vi "Practice with Arrays.vi"() -> ()   [LabVIEW 2016]
panel:
  out "y":dbl[](array[numeric])
  out "x-y":dbl[](array[numeric])
  out "x":dbl[](array[numeric])
  in  "Input Array":dbl[](array[numeric])
  in  "Input element":dbl
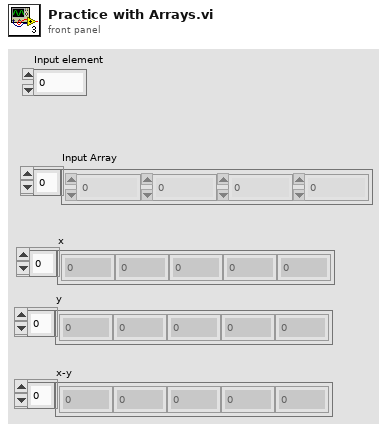
[diagram p1: front panel]
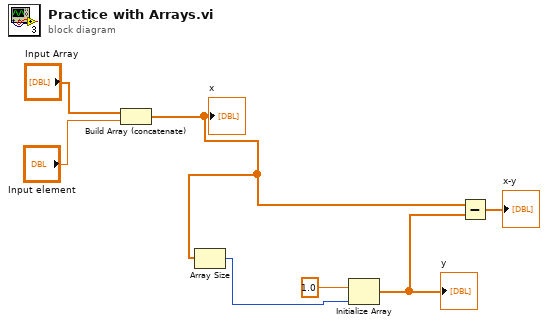
[diagram p0: block diagram]
diagram:
  n1 = Build Array (concatenate)("Input Array", "Input element") -> (w3:dbl[])
  "x" <- w3
  n2 = Array Size(array=w3) -> (size(s)=w4:i32)
  n3 = Initialize Array(1.0 ("元素"), w4) -> (w1:dbl[])
  "y" <- w1
  n4 = Subtract(x=w3, y=w1) -> (x-y=→"x-y":dbl[])
